vi "Module Type.vi"(11 "Hardware Info Module in":refnum<class "Hardware Info Module.lvclass">) -> (2 "Module Type":string)   [LabVIEW 2020, in "Volatus.lvlib" / "Hardware Info Module.lvclass"]
uses:
  Hardware Info Module.lvclass
  Hardware Info Module.lvclass/Hardware Info Module.ctl
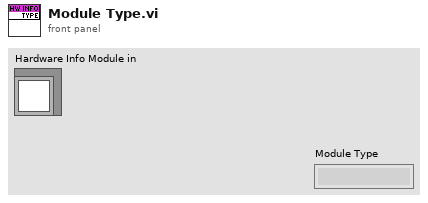
[diagram p1: front panel]
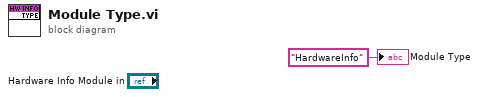
[diagram p0: block diagram]
diagram:
  "Module Type" <- "HardwareInfo" ("Module Type")
